vi "XL320_Scan for Motors.vi"(0 "VISA resource name":refnum<visa-resource-name>, 5 "Starting ID (0)":u8, 7 "Ending ID (252)":u8=252, 9 "Search Timeout (10000 ms)":u32=10000, 11 "error in (no error)":errorcluster) -> (4 "VISA resource name out":refnum<visa-resource-name>, 6 "Motors IDs Found":u8[](array[numeric]), 15 "error out":errorcluster)   [LabVIEW 2017, in "Dynamixel XL320.lvlib"]
doc: "Scans sequentially for motors between <b>Starting ID</b> and <b>Ending ID</b> for no longer than <b>Search Timeout</b>. If all of the motors do not have unique IDs, then motors with duplicate IDs may not be found."
uses:
  <instrlib>/Dynamixel XL320 (Drivers instrument)/Dynamixel XL320.lvlib
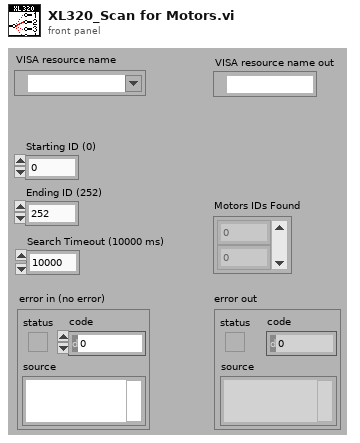
[diagram p1: front panel]
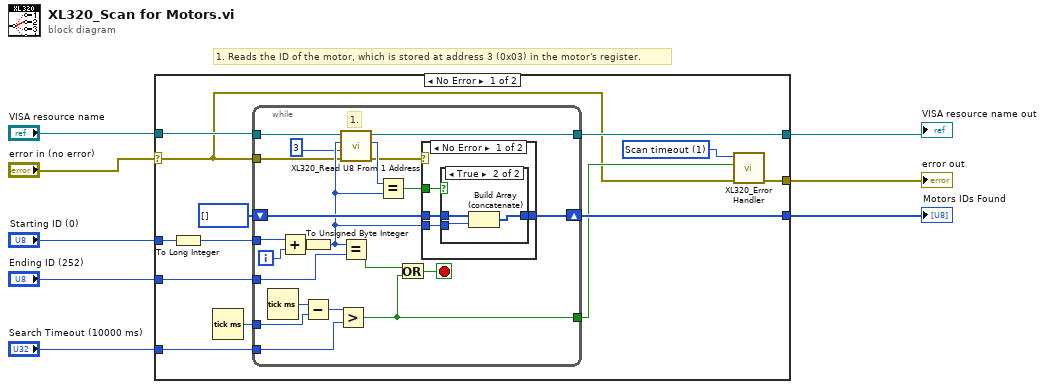
[diagram p0: block diagram]
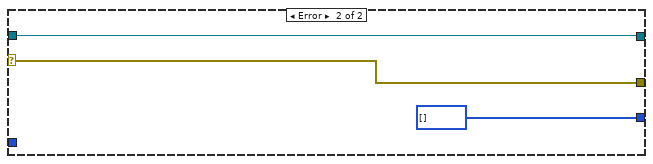
[diagram p4: hidden frame]
diagram:
  # "1. Reads the ID of the motor, which is stored at address 3 (0x03) in the motor's register."
  n1 = case shown="No Error" "error in (no error)" {
    selector: "error in (no error)" -> [w10 w54]
    tunnel: "VISA resource name" -> [w15 w53]
    tunnel: [w21 w53] -> w2
    tunnel: [w9 w54] -> w3
    tunnel: [w17 u8[] []] -> w8
    tunnel: "Starting ID (0)" -> [w20 _]
    tunnel: "Ending ID (252)" -> [w18 _]
    tunnel: "Search Timeout (10000 ms)" -> [w13 _]
    frame No Error {
      w12 = u16 1 items=["Default (no error)", "Scan timeout", "Invalid motor checksum", "Unexpected return string", "Invalid address range"] ("Error type")
      n2 = To Long Integer(number=w20) -> (32bit integer=w16:i32)
      n3 = Tick Count (ms)() -> (millisecond timer value=w14:u32)
      n4 = while {
        tunnel: w15 -> [w28]
        shift-right: [w38] -> w17
        shift-left: u8[] [] -> [w40]
        tunnel: [w24] -> w21
        tunnel: w10 -> [w25]
        tunnel: w16 -> [w36]
        tunnel: w18 -> [w35]
        tunnel: w14 -> [w32]
        tunnel: w13 -> [w30]
        tunnel: [w29] -> w11
        i -> [w42]
        stop <- w37 stop-if-true
        # "1."
        n5 = Tick Count (ms)() -> (millisecond timer value=w33:u32)
        n6 = Add(x=w36, y=w42) -> (x+y=w39:i32)
        n7 = To Unsigned Byte Integer(number=w39) -> (unsigned 8bit integer=w27:u8)
        n8 = Subtract(x=w33, y=w32) -> (x-y=w31:u32)
        n9 = Greater?(x=w31, y=w30) -> (0:w29:bool)
        n10 = call <instrlib>:"XL320_Read U8 From 1 Address.vi"("Error in (no error)"=w25, "Address number (0)"=u16 3, "Motor ID (0)"=w27, "VISA resource name"=w28) -> ("error out"=w22:errorcluster, "Data"=w23:u8, "VISA resource name out"=w24:refnum<visa-resource-name>)  [unwired: 5 in]
        n11 = Equal?(x=w27, y=w35) -> (x = y?=w34:bool)
        n12 = Equal?(x=w23, y=w27) -> (x = y?=w41:bool)
        n13 = Or(x=w34, y=w29) -> (x .or. y?=w37:bool)
        n14 = case shown="No Error" w22 {
          tunnel: w41 -> [w46 _]
          tunnel: w40 -> [w45 w51]
          tunnel: [w44 w51] -> w38
          tunnel: w27 -> [w43 _]
          frame No Error {
            n15 = case shown="True" w46 {
              tunnel: w45 -> [w47 w50]
              tunnel: w43 -> [_ w49]
              tunnel: [w47 w48] -> w44
              frame False {
              }
              frame True {
                n16 = Build Array (concatenate)(w50, w49) -> (w48:u8[])
              }
            }
          }
          frame Error {
          }
        }
      }
      n17 = call <instrlib>:"XL320_Error Handler.vi"("error in (no error)"=w10, "Error? (no error)"=w11, "Error type"=w12) -> ("error out"=w9:errorcluster)  [unwired: 8 in]
    }
    frame Error {
    }
  }
  "Motors IDs Found" <- w8
  "error out" <- w3
  "VISA resource name out" <- w2
